vi "生成校准信息.vi"(5 "量程选择":enum16{"低量程", "高量程"}(ring), 7 "公式系数":cluster{"K":string, "B":string, "X^2":string}, 8 "启用":bool[](array[boolean]), 9 "校准时间":string[](array[string]), 10 "信号值":string[](array[string]), 11 "校准浓度":string[](array[string])) -> ()   [LabVIEW 2016, in "斯坦道CODMn.lvlib"]
panel:
  out "data":T1
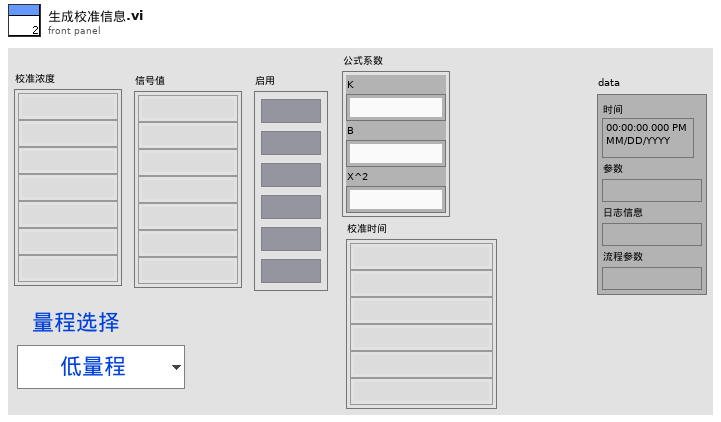
[diagram p1: front panel]
types:
  T1 = typedef "操作日志字段定义.ctl" = cluster{"时间":timestamp, "参数":string, "日志信息":string, "流程参数":string}
  T2 = cluster{"时间标识":timestamp, "参数":string, "日志信息":string, "流程参数":string}
  T3 = typedef "数据库类型.ctl" = enum16{"Access", "SQLite"}
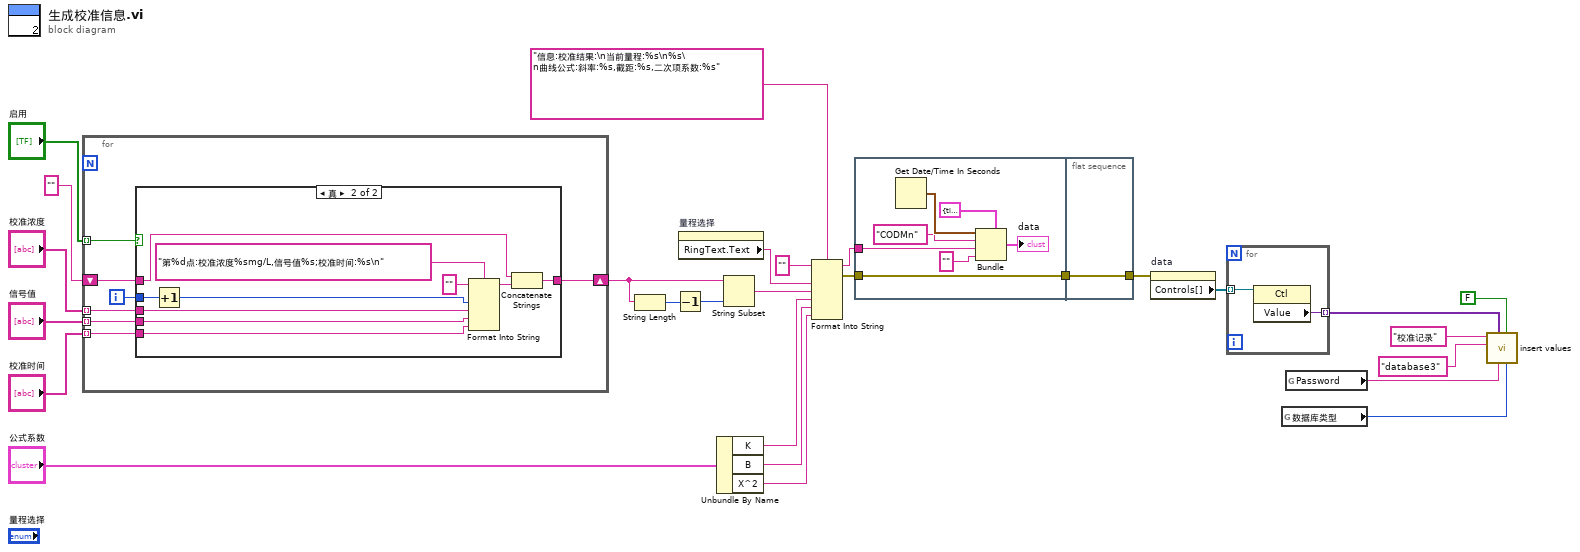
[diagram p0: block diagram]
diagram:
  n1 = for {
    tunnel: "启用" -> [w34] mode=indexing
    tunnel: "校准浓度" -> [w32] mode=indexing
    tunnel: "信号值" -> [w31] mode=indexing
    shift-right: [w30] -> w21
    shift-left: "" -> [w29]
    tunnel: "校准时间" -> [w28] mode=indexing
    i -> [w33]
    n2 = case shown="真" w34 {
      tunnel: w33 -> [_ w43]
      tunnel: w32 -> [_ w42]
      tunnel: w31 -> [_ w41]
      tunnel: [w35 w38] -> w30
      tunnel: w29 -> [w35 w37]
      tunnel: w28 -> [_ w36]
      frame False {
      }
      frame True {
        n3 = Increment(x=w43) -> (x+1=w44:i32)
        n4 = Format Into String(format string="第%d点:校准浓度%smg/L,信号值%s;校准时间:%s\n" ("格式字符串"), initial string="" ("初始字符串"), w44, w42, w41, w36) -> (resulting string=w39:string)  [unwired: 1 in, 1 out]
        n5 = Concatenate Strings(w37, w39) -> (w38:string)
      }
    }
  }
  n6 = String Length(string=w21) -> (length=w20:i32)
  n7 = Decrement(x=w20) -> (x-1=w19:i32)
  n8 = property on="量程选择" class="Enum (严格)"() -> ("RingText.Text"=w12:string)  [unwired: 2 in, 2 out]
  n9 = Unbundle By Name("公式系数") -> ("K"=w16:string, "B"=w15:string, "X^2"=w14:string)
  n10 = String Subset(string=w21, length (rest)=w19) -> (substring=w13:string)  [unwired: 1 in]
  n11 = Format Into String(format string="信息:校准结果:\n当前量程:%s\n%s\n曲线公式:斜率:%s,截距:%s,二次项系数:%s", initial string="" ("初始字符串"), w12, w13, w16, w15, w14) -> (resulting string=w6:string, error out=w2:errorcluster)  [unwired: 1 in]
  n12 = flat-sequence {
    tunnel: w6 -> [w48]
    tunnel: [w46] -> w3
    tunnel: w2 -> [w46]
    tunnel: w3 -> [w53]
    tunnel: [w53] -> w1
    frame #0 {
      n13 = Get Date/Time In Seconds() -> (seconds since 1Jan1904=w50:timestamp)
      n14 = Bundle(cluster=T2 {"时间标识"=timestamp(0 s since 1904-01-01), "参数"="", "日志信息"="", "流程参数"=""} ("data in"), "时间标识"=w50, "参数"="CODMn" ("table输入"), "日志信息"=w48, "流程参数"="" ("table输入")) -> (→"data":T2)
    }
    frame #1 {
    }
  }
  n15 = property on="data" class="Clust (严格)"(error in=w1) -> ("Controls[]"=w7:refnum<vi>[])  [unwired: 1 in, 2 out]
  n16 = for {
    tunnel: w7 -> [w55] mode=indexing
    tunnel: [w54] -> w11 mode=indexing
    n17 = property class="Ctl"(reference=w55) -> ("Value"=w54:variant)  [unwired: 1 in, 2 out]
  }
  n18 = global read "CODMn断电保存全局变量.vi" "数据库类型"() -> (w4:T3)
  n19 = global read "CODMn断电保存全局变量.vi" "Password"() -> (w5:string)
  n20 = call "insert values.vi"("数据库类型"=w4, "是否创建唯一键"=FALSE, "Password"=w5, "data"=w11, "database"="database3", "Tabe Name"="校准记录") -> ()  [unwired: 5 in, 1 out]
